vi "FilterRudder.vi"(9 "Queue timeout (ms)":i32=200, 10 "NotifierReff 2":T1, 11 "Queue in":refnum<queue>) -> ()   [LabVIEW 2013]
uses:
  Data/TypeDefs/Notifiers.ctl
  Data/TypeDefs/UTM Location.ctl
  Data/TypeDefs/GPS Sensor Status.ctl
  Data/TypeDefs/Sail Set Suggestions.ctl
  Data/TypeDefs/Rudder Set Suggestions.ctl
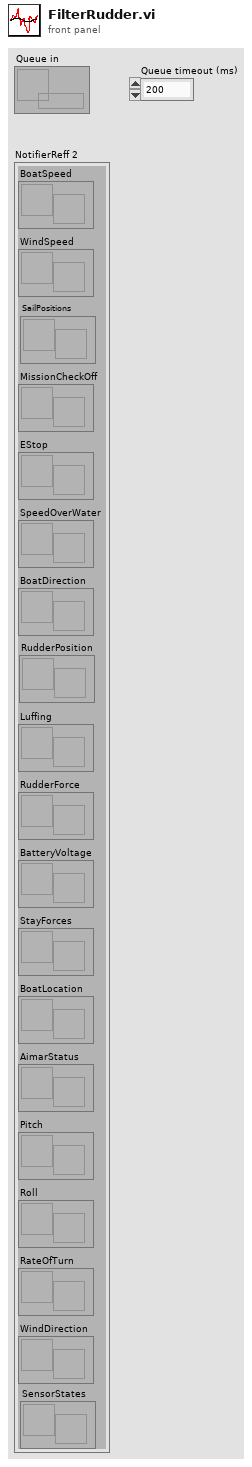
[diagram p1: front panel]
types:
  T1 = typedef "Notifiers.ctl" = cluster{"BoatSpeed":refnum<notifier>, "WindSpeed":refnum<notifier>, "MissionCheckOff":refnum<notifier>, "EStop":refnum<notifier>, "SpeedOverWater":refnum<notifier>, "BoatDirection":refnum<notifier>, "Luffing":refnum<notifier>, "RudderForce":refnum<notifier>, "BatteryVoltage":refnum<notifier>, "StayForces":refnum<notifier>, "BoatLocation":refnum<notifier>, "AimarStatus":refnum<notifier>, "Pitch":refnum<notifier>, "Roll":refnum<notifier>, "RateOfTurn":refnum<notifier>, "WindDirection":refnum<notifier>, "SailPositions":refnum<notifier>, "RudderPosition":refnum<notifier>, "SensorStates":refnum<notifier>}
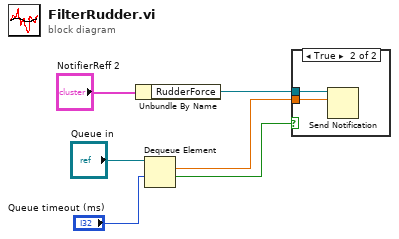
[diagram p0: block diagram]
diagram:
  n1 = Unbundle By Name("NotifierReff 2") -> ("RudderForce"=w3:refnum<notifier>)
  n2 = Dequeue Element(queue="Queue in", timeout in ms (-1)="Queue timeout (ms)") -> (element=w6:dbl, timed out?=w1:bool)  [unwired: 1 in, 2 out]
  n3 = case shown="True" w1 {
    tunnel: w6 -> [_ w8]
    tunnel: w3 -> [_ w7]
    frame False {
    }
    frame True {
      n4 = Send Notification(notification=w8, notifier=w7) -> ()  [unwired: 1 in, 2 out]
    }
  }
